vi "ElevBaseModeToDash.vi"(10 "Update?":bool, 11 "ElevBasePosIn":T1) -> (3 "ElevBasePosOut":T1)   [LabVIEW 2018]
uses:
  ElevBasePos.ctl
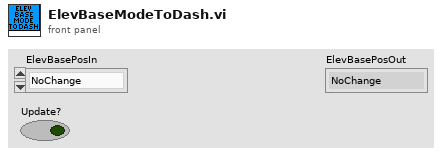
[diagram p1: front panel]
types:
  T1 = typedef "ElevBasePos.ctl" = enum16{"NoChange", "ShipHatch", "RocketHatch", "Carry", "Cargo"}
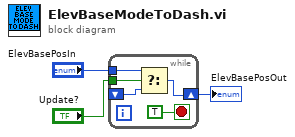
[diagram p0: block diagram]
diagram:
  n1 = while {
    tunnel: "Update?" -> [w8]
    tunnel: "ElevBasePosIn" -> [w7]
    shift-right: [w6] -> w1
    shift-left: _ -> [w5]
    stop <- TRUE stop-if-true
    n2 = Select(t=w7, s=w8, f=w5) -> (s? t:f=w6:T1)
  }
  "ElevBasePosOut" <- w1
